vi "Read Measurement Timeout (ms).vi"(8 "error in (no error)":errorcluster, 11 "ExperimentVariables in":refnum<class "ExperimentVariables.lvclass">) -> (0 "error out":errorcluster, 2 "Measurement Timeout (ms)":u32=1, 3 "ExperimentVariables out":refnum<class "ExperimentVariables.lvclass">)   [LabVIEW 2013, in "ExperimentVariables.lvclass"]
uses:
  ExperimentVariables.lvclass
  ExperimentVariables.lvclass/ExperimentVariables.ctl
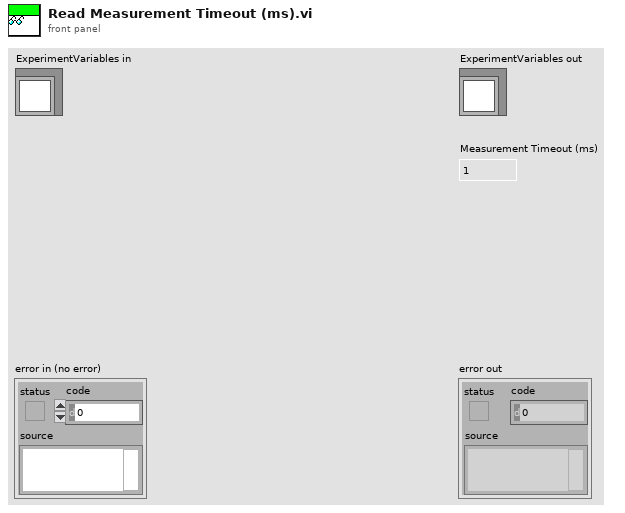
[diagram p1: front panel]
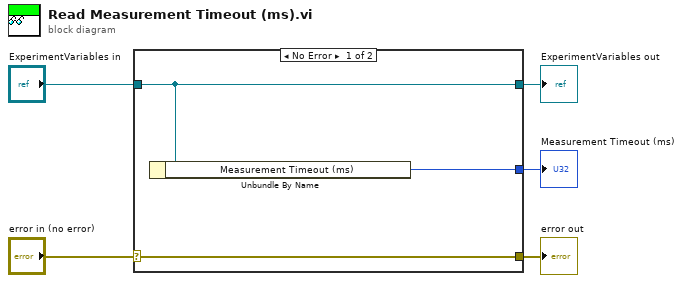
[diagram p0: block diagram]
diagram:
  n1 = case shown="No Error" "error in (no error)" {
    selector: "error in (no error)" -> [w8 w9]
    tunnel: [w8 w9] -> w4
    tunnel: [w7 w10] -> w2
    tunnel: "ExperimentVariables in" -> [w7 w10]
    tunnel: [w6 _] -> w1
    frame No Error {
      n2 = Unbundle By Name(w7) -> ("Measurement Timeout (ms)"=w6:u32)
    }
    frame Error {
    }
  }
  "error out" <- w4
  "ExperimentVariables out" <- w2
  "Measurement Timeout (ms)" <- w1
